vi "Write Result and Failures.vi"(4 "Vacuum?":bool, 5 "Leak":bool, 6 "Test Configuration":T1, 7 "Func":bool, 8 "error in (no error)":errorcluster, 11 "Step":i32) -> (0 "error out":errorcluster)   [LabVIEW 2015]
uses:
  Controls/Test Configuration.ctl
  Controls/Vacuum Test.ctl
  Controls/Test Timing.ctl
  Controls/Vaccum Thresholds.ctl
  Controls/Helium Test.ctl
  Controls/Helium Thresholds.ctl
  Controls/Functional Test.ctl
  User Interface/UI Handler/UI Handler.lvclass
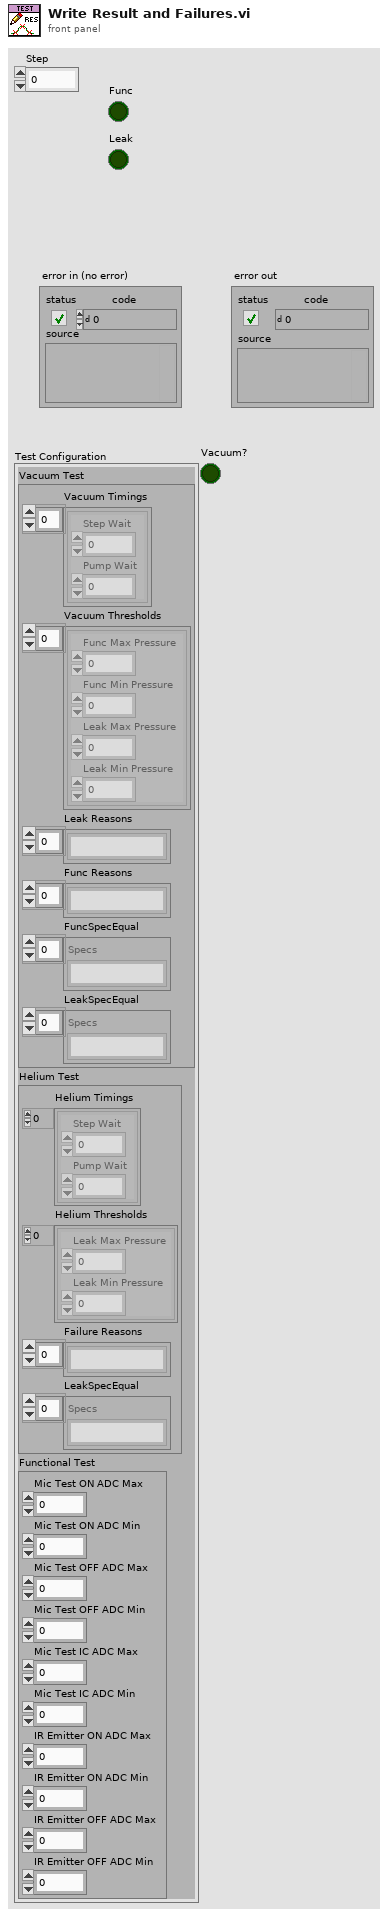
[diagram p1: front panel]
types:
  T1 = typedef "Test Configuration.ctl" = cluster{"Vacuum Test":T2, "Helium Test":T5, "Functional Test":T7}
  T2 = typedef "Vacuum Test.ctl" = cluster{"Vacuum Timings":T3[], "Vacuum Thresholds":T4[], "Leak Reasons":string[], "Func Reasons":string[], "FuncSpecEqual":string[], "LeakSpecEqual":string[]}
  T3 = typedef "Test Timing.ctl" = cluster{"Step Wait":dbl, "Pump Wait":dbl}
  T4 = typedef "Vaccum Thresholds.ctl" = cluster{"Func Max Pressure":dbl, "Func Min Pressure":dbl, "Leak Max Pressure":dbl, "Leak Min Pressure":dbl}
  T5 = typedef "Helium Test.ctl" = cluster{"Helium Timings":T3[], "Helium Thresholds":T6[], "Failure Reasons":string[], "LeakSpecEqual":string[]}
  T6 = typedef "Helium Thresholds.ctl" = cluster{"Leak Max Pressure":dbl, "Leak Min Pressure":dbl}
  T7 = typedef "Functional Test.ctl" = cluster{"Mic Test ON ADC Max":dbl, "Mic Test ON ADC Min":dbl, "Mic Test OFF ADC Max":dbl, "Mic Test OFF ADC Min":dbl, "Mic Test IC ADC Max":dbl, "Mic Test IC ADC Min":dbl, "IR Emitter ON ADC Max":dbl, "IR Emitter ON ADC Min":dbl, "IR Emitter OFF ADC Max":dbl, "IR Emitter OFF ADC Min":dbl}
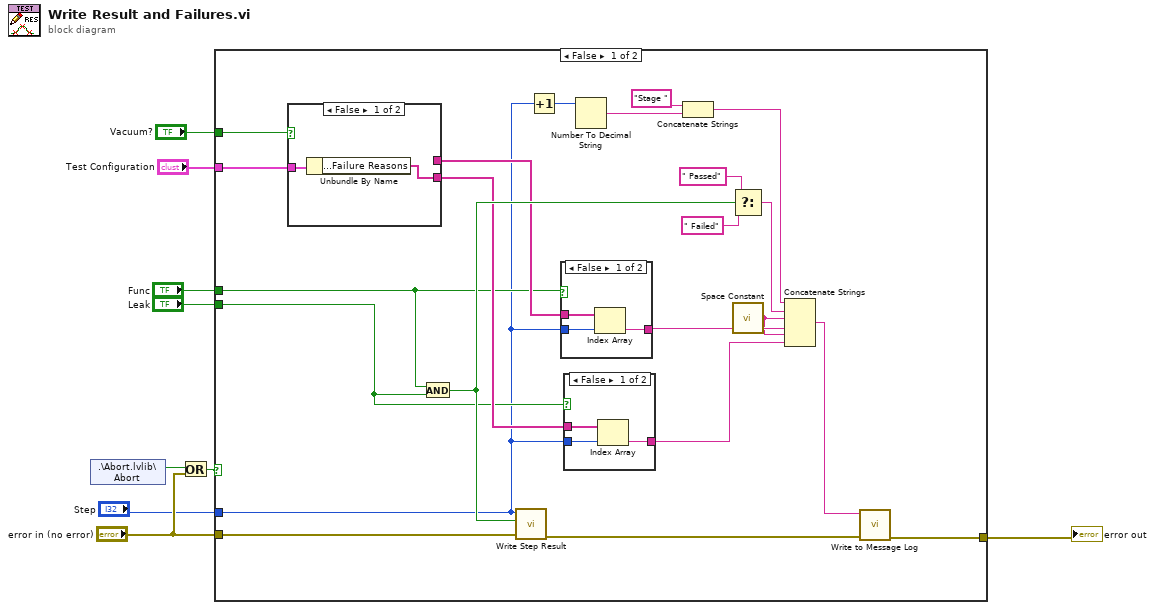
[diagram p0: block diagram]
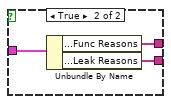
[diagram p2: hidden frame]
diagram:
  n1 = shared-variable ".\\Abort.lvlib\\Abort"() -> (w8:bool)  [unwired: 1 in, 1 out]
  n2 = Or(x=w8, y="error in (no error)") -> (x .or. y?=w6:bool)
  n3 = case shown="False" w6 {
    tunnel: [w31 w43] -> w9
    tunnel: "error in (no error)" -> [w30 w43]
    tunnel: "Test Configuration" -> [w14 _]
    tunnel: "Func" -> [w13 _]
    tunnel: "Leak" -> [w12 _]
    tunnel: "Step" -> [w11 _]
    tunnel: "Vacuum?" -> [w10 _]
    frame False {
      n4 = case shown="False" w10 {
        tunnel: [_ w36] -> w22
        tunnel: [w32 w35] -> w21
        tunnel: w14 -> [w33 w34]
        frame False {
          n5 = Unbundle By Name(w33) -> ("Helium Test.Failure Reasons"=w32:string[])
        }
        frame True {
          n6 = Unbundle By Name(w34) -> ("Vacuum Test.Func Reasons"=w36:string[], "Vacuum Test.Leak Reasons"=w35:string[])
        }
      }
      n7 = And(x=w13, y=w12) -> (x .and. y?=w23:bool)
      n8 = call "Write Step Result.vi"("error in (no error)"=w30, "Pass?"=w23, "Step Index"=w11) -> ("error out"=w29:errorcluster)  [unwired: 8 in]
      n9 = Increment(x=w11) -> (x+1=w19:i32)
      n10 = case shown="False" w13 {
        tunnel: w22 -> [w42 _]
        tunnel: w11 -> [w41 _]
        tunnel: [w40 _] -> w26
        frame False {
          n11 = Index Array(array=w42, index=w41) -> (element=w40:string)
        }
        frame True {
        }
      }
      n12 = case shown="False" w12 {
        tunnel: w21 -> [w39 _]
        tunnel: w11 -> [w38 _]
        tunnel: [w37 _] -> w24
        frame False {
          n13 = Index Array(array=w39, index=w38) -> (element=w37:string)
        }
        frame True {
        }
      }
      n14 = Number To Decimal String(number=w19) -> (decimal integer string=w17:string)  [unwired: 1 in]
      n15 = Concatenate Strings("Stage " ("string"), w17) -> (w15:string)
      n16 = Select(t=" Passed", s=w23, f=" Failed") -> (s? t:f=w27:string)
      n17 = call <vilib>:"Space Constant.vi"() -> ("String"=w25:string)
      n18 = Concatenate Strings(w15, w27, w25, w26, w25, w24) -> (w20:string)
      n19 = call "Write to Message Log.vi"("error in (no error)"=w29, "Message"=w20) -> ("error out"=w31:errorcluster)  [unwired: 9 in]
    }
    frame True {
    }
  }
  "error out" <- w9
